vi "MakeMaze.vi"(8 "error in (no error)":errorcluster, 11 "MazeGame in":refnum<class "MazeGame.lvclass">) -> (0 "error out":errorcluster, 2 "Maze":refnum<class "Maze.lvclass">, 3 "MazeGame out":refnum<class "MazeGame.lvclass">)   [LabVIEW 2020, in "FactoryMethod.lvlib" / "NoParametrizedFactoryMethod.lvlib" / "MazeGame.lvclass"]
uses:
  MazeGame.lvclass
  GoFcommonClasses/Maze/Maze.lvclass
  MazeGame.lvclass/MazeGame.ctl
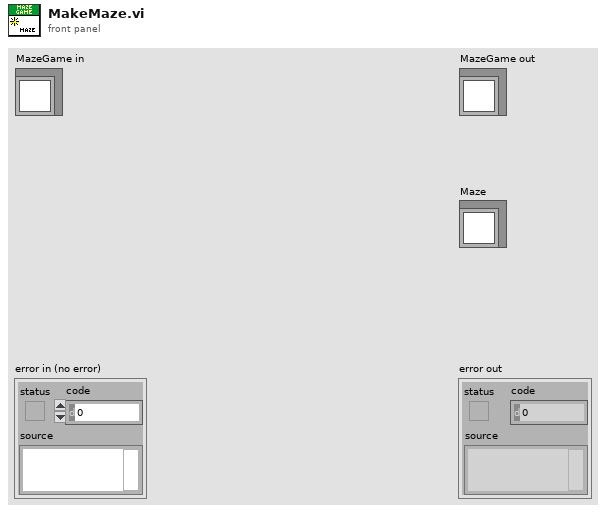
[diagram p1: front panel]
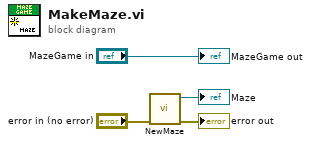
[diagram p0: block diagram]
diagram:
  n1 = call "NewMaze.vi"("error in (no error)"="error in (no error)") -> ("error out"=→"error out":errorcluster, "Maze"=→"Maze":refnum<class "Maze.lvclass">)  [unwired: 9 in]
  "MazeGame out" <- "MazeGame in"
